vi "SetMotorInfoProperties.vi"(9 "data":T2, 10 "data event properties in":T1[](array[typedef])) -> (2 "data event properties out":T1[](array[typedef]))   [LabVIEW 2017, in "McsaDataEventCreator.lvlib"]
uses:
  <vilib>/addons/InsightCM/Devices/Shared/Mcsa/McsaDataEventCreator/McsaDataEventCreator.lvlib
  <vilib>/addons/InsightCM/MessageBus/Base/controls/KeyValuePair.ctl
  <vilib>/addons/InsightCM/Devices/Shared/Common/DataFlow/controls/Data.ctl
  <vilib>/addons/InsightCM/Utilities/DataAccessors/controls/wfmSGL_DVR.ctl
  <vilib>/addons/PointValueMap/controls/PointMap.ctl
  <vilib>/addons/InsightCM/Devices/Shared/Common/DataFlow/controls/Type.ctl
  <vilib>/addons/InsightCM/Utilities/MCSA/McsaUtilities.lvlib
  <vilib>/addons/PointValueMap/PointValueMap.lvlib
  <vilib>/addons/InsightCM/Devices/Shared/Common/DataFlow/DataFlow.lvlib
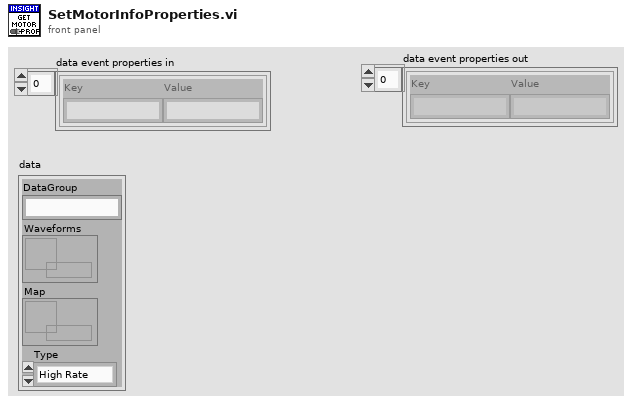
[diagram p1: front panel]
types:
  T1 = typedef "KeyValuePair.ctl" = cluster{"Key":string, "Value":string}
  T2 = typedef "DataFlow.lvlib/Data.ctl" = cluster{"DataGroup":string, "Waveforms":T3, "Map":T4, "Type":T5}
  T3 = typedef "wfmSGL_DVR.ctl" = refnum<data-value>
  T4 = typedef "PointValueMap.lvlib/PointMap.ctl" = refnum<data-value>
  T5 = typedef "DataFlow.lvlib/Type.ctl" = enum16{"High Rate", "Low Rate", "Burst Mode"}
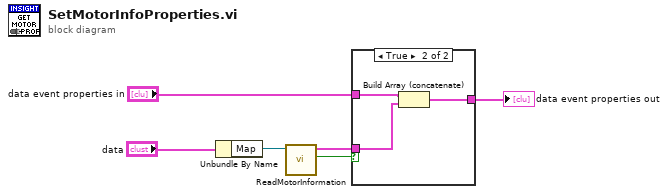
[diagram p0: block diagram]
diagram:
  n1 = Unbundle By Name("data") -> ("Map"=w3:T4)
  n2 = call <vilib>:"ReadMotorInformation.vi"("Map"=w3) -> ("found"=w1:bool, "Properties"=w2:T1[])  [unwired: 8 in, 1 out]
  n3 = case shown="True" w1 {
    tunnel: "data event properties in" -> [w7 w10]
    tunnel: [w7 w9] -> w4
    tunnel: w2 -> [_ w8]
    frame False {
    }
    frame True {
      n4 = Build Array (concatenate)(w10, w8) -> (w9:T1[])
    }
  }
  "data event properties out" <- w4
